vi "read_params.vi"(8 "error in (no error)":errorcluster caption="entrée d'erreur (pas d'erreur)", 11 "SGDRegressor en entrée":refnum<class "SGDRegressor.lvclass">) -> (0 "error out":errorcluster caption="sortie d'erreur", 2 "params":T1={"loss"="squared_loss", "penalty"="l2", "alpha"=0.0001, "l1_ratio"=0.15, "fit_intercept"=TRUE, "max_iter"=1000.0, "tol"=0.001, "shuffle"=TRUE, "verbose"=0.0, "epsilon"=0.1, "random_state"=0.0, "learning_rate"="invscaling", "eta0"=0.01, "power_t"=0.25, "early_stopping"=FALSE, "validation_fraction"=0.1, "n_iter_no_change"=5.0, "warm_start"=FALSE, "average"={"average_type"="bool", "average_bool"=FALSE, "average_int"=0.0}}, 3 "SGDRegressor en sortie":refnum<class "SGDRegressor.lvclass">)   [LabVIEW 2020, in "SGDRegressor.lvclass"]
uses:
  SGDRegressor.lvclass
  Controls/sgdregressor_params.ctl
  SGDRegressor.lvclass/SGDRegressor.ctl
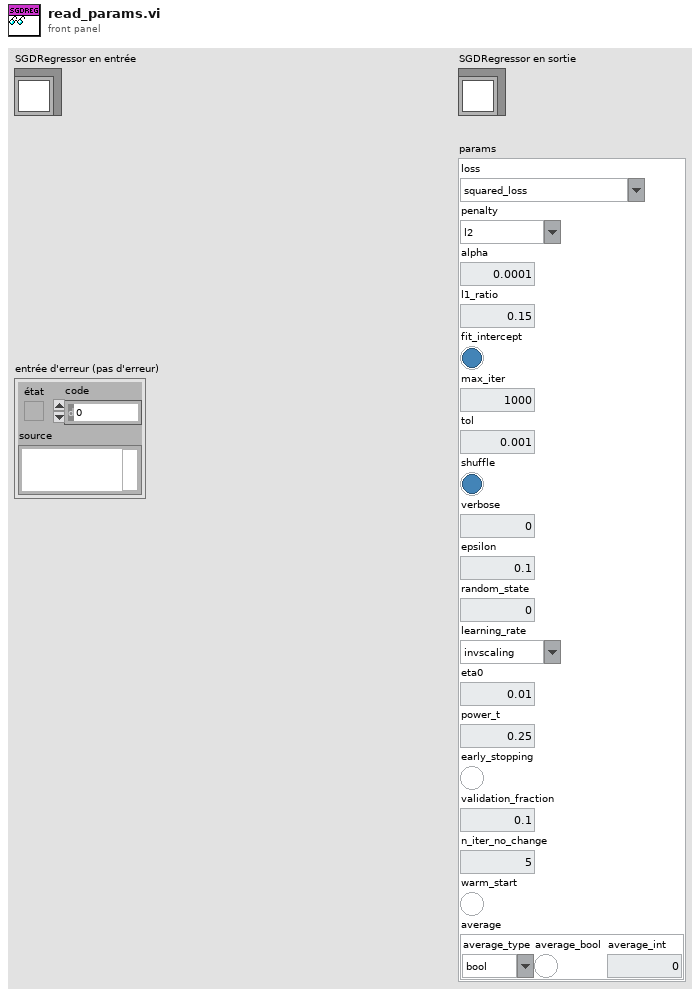
[diagram p1: front panel]
types:
  T1 = typedef "sgdregressor_params.ctl" = cluster{"loss":string, "penalty":string, "alpha":dbl, "l1_ratio":dbl, "fit_intercept":bool, "max_iter":dbl, "tol":dbl, "shuffle":bool, "verbose":dbl, "epsilon":dbl, "random_state":dbl, "learning_rate":string, "eta0":dbl, "power_t":dbl, "early_stopping":bool, "validation_fraction":dbl, "n_iter_no_change":dbl, "warm_start":bool, "average":cluster{"average_type":string, "average_bool":bool, "average_int":dbl}}
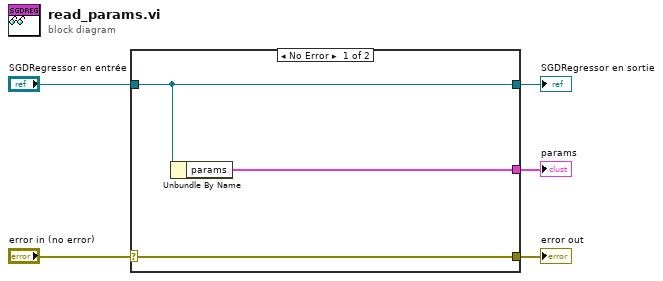
[diagram p0: block diagram]
diagram:
  n1 = case shown="No Error" "error in (no error)" {
    selector: "error in (no error)" -> [w8 w9]
    tunnel: [w8 w9] -> w4
    tunnel: [w7 w10] -> w2
    tunnel: "SGDRegressor en entrée" -> [w7 w10]
    tunnel: [w6 _] -> w1
    frame No Error {
      n2 = Unbundle By Name(w7) -> ("params"=w6:T1)
    }
    frame Error {
    }
  }
  "error out" <- w4
  "SGDRegressor en sortie" <- w2
  "params" <- w1
